vi "Query Multi Eval Meas List Segment DMRS Type A.vi"(6 "Segment (1)":T3=1, 7 "Bandwidth Part (BWP0)":T1 items=["BWP0"], 8 "error in (no error)":errorcluster, 9 "Carrier Component (1)":T2=1, 10 "Instance (1)":T4=1, 11 "VISA resource name":refnum<visa-resource-name>) -> (0 "error out":errorcluster, 1 "Max Length":i32=1, 2 "Additional Position":i32, 3 "VISA resource name out":refnum<visa-resource-name>, 4 "Config Type":i32=1)   [LabVIEW 2015, in "Rohde&Schwarz CMXP NR FR2 Measurement.lvlib"]
doc: "Configures the DM-RS for mapping type A. The settings apply to the <BWP> on carrier <cc> in segment <no>.\n\nAttribute:\n-\n\nRemote-control command:\nCONFigure:NRMMw:MEAS<i>:LIST:SEGMent<no>[:CC<cc>]:BWPart:PUSCh:DMTA? <BWP>"
uses:
  <instrlib>/Rohde&Schwarz CMXP NR FR2 Measurement/Rohde&Schwarz CMXP NR FR2 Measurement.lvlib
  <instrlib>/Rohde&Schwarz CMXP NR FR2 Measurement/Private/_Instance.ctl
  <instrlib>/Rohde&Schwarz CMXP NR FR2 Measurement/Private/_Segment.ctl
  <instrlib>/Rohde&Schwarz CMXP NR FR2 Measurement/Private/_Carrier Component.ctl
  <instrlib>/Rohde&Schwarz CMXP NR FR2 Measurement/Private/_Bandwidth Part.ctl
  <instrlib>/Rohde&Schwarz CMXP NR FR2 Measurement/Private/rsidr_core.llb/rsidr_core.lvlib
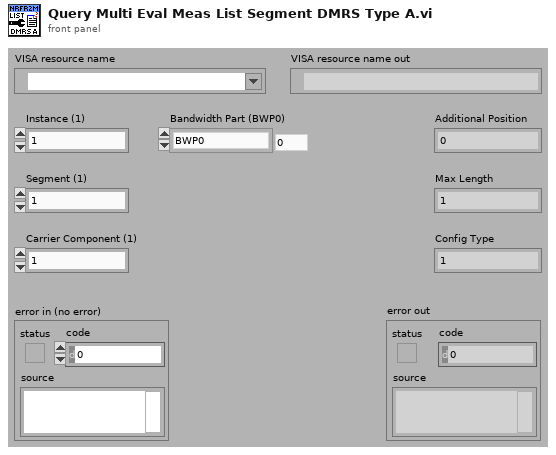
[diagram p1: front panel]
types:
  T1 = typedef "Rohde&Schwarz CMXP NR FR2 Measurement.lvlib/_Bandwidth Part.ctl" = i32
  T2 = typedef "Rohde&Schwarz CMXP NR FR2 Measurement.lvlib/_Carrier Component.ctl" = i32
  T3 = typedef "Rohde&Schwarz CMXP NR FR2 Measurement.lvlib/_Segment.ctl" = i32
  T4 = typedef "Rohde&Schwarz CMXP NR FR2 Measurement.lvlib/_Instance.ctl" = i32
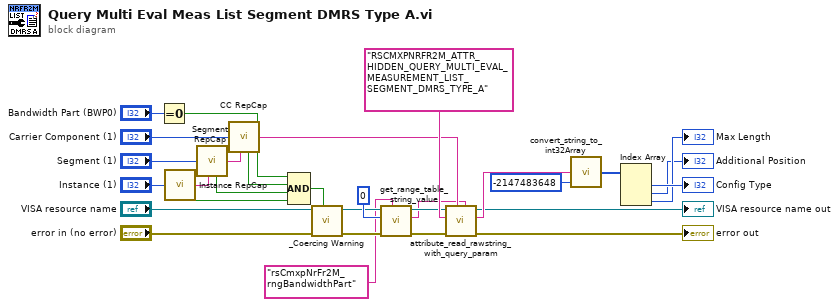
[diagram p0: block diagram]
diagram:
  n1 = Equal To 0?(x="Bandwidth Part (BWP0)") -> (x = 0?=w5:bool)
  n2 = call <instrlib>:"Instance RepCap.vi"("Instance In"="Instance (1)") -> ("In Range?"=w24:bool, "RepCap Identifier Out"=w3:string)  [unwired: 1 in]
  n3 = call <instrlib>:"Segment RepCap.vi"("Segment In"="Segment (1)", "RepCap String In (\"\")"=w3) -> ("In Range?"=w23:bool, "RepCap Identifier Out"=w22:string)
  n4 = call <instrlib>:"CC RepCap.vi"("CC In"="Carrier Component (1)", "RepCap String In (\"\")"=w22) -> ("In Range?"=w21:bool, "RepCap Identifier Out"=w10:string)
  n5 = Compound Arithmetic op=AND(w5, w21, w23, w24) -> (w27:bool)
  n6 = call <instrlib>:"_Coercing Warning.vi"("In Range?"=w27, "error in (no error)"="error in (no error)", "VISA resource name"="VISA resource name") -> ("error out"=w19:errorcluster, "VISA resource name out"=w18:refnum<visa-resource-name>)  [unwired: 7 in]
  n7 = call <instrlib>:"get_range_table_string_value.vi"("Range Table ID in"="rsCmxpNrFr2M_rngBandwidthPart", "error in"=w19, "I32 input"=0, "VISA resource name"=w18) -> ("error out"=w12:errorcluster, "String Value out"=w9:string, "VISA resource name out"=w11:refnum<visa-resource-name>)  [unwired: 5 in]
  n8 = call <instrlib>:"attribute_read_rawstring_with_query_param.vi"("Query Parameter (None)"=w9, "Repeated Capability"=w10, "error in"=w12, "Attribute ID"="RSCMXPNRFR2M_ATTR_HIDDEN_QUERY_MULTI_EVAL_MEASUREMENT_LIST_SEGMENT_DMRS_TYPE_A", "VISA resource name"=w11) -> ("error out"=→"error out":errorcluster, "Raw String out"=w15:string, "VISA resource name out"=→"VISA resource name out":refnum<visa-resource-name>)  [unwired: 4 in]
  n9 = call <instrlib>:"convert_string_to_int32Array.vi"("default (0)"=-2147483648, "string in"=w15) -> ("int32 array out"=w14:i32[])  [unwired: 2 in, 1 out]
  n10 = Index Array(array=w14) -> (element #1=→"Config Type":i32, element #2=→"Additional Position":i32, element #3=→"Max Length":i32)  [unwired: 3 in]
